vi "Query Error Status.vi"(8 "error in (no error)":errorcluster, 11 "VISA resource name":refnum<visa-resource-name>) -> (0 "error out":errorcluster, 2 "Error Status Data Message":string, 3 "VISA resource name out":refnum<visa-resource-name>)   [LabVIEW 2020, in "Stanford Research SR865.lvlib"]
doc: "Queries the Error Status register for the Error Data Register group. Essentially, it is used to observe possible invalid results."
uses:
  Stanford Research SR865.lvlib
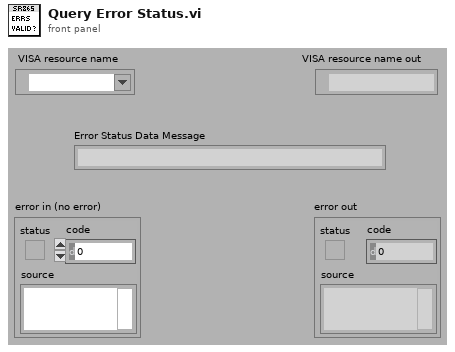
[diagram p1: front panel]
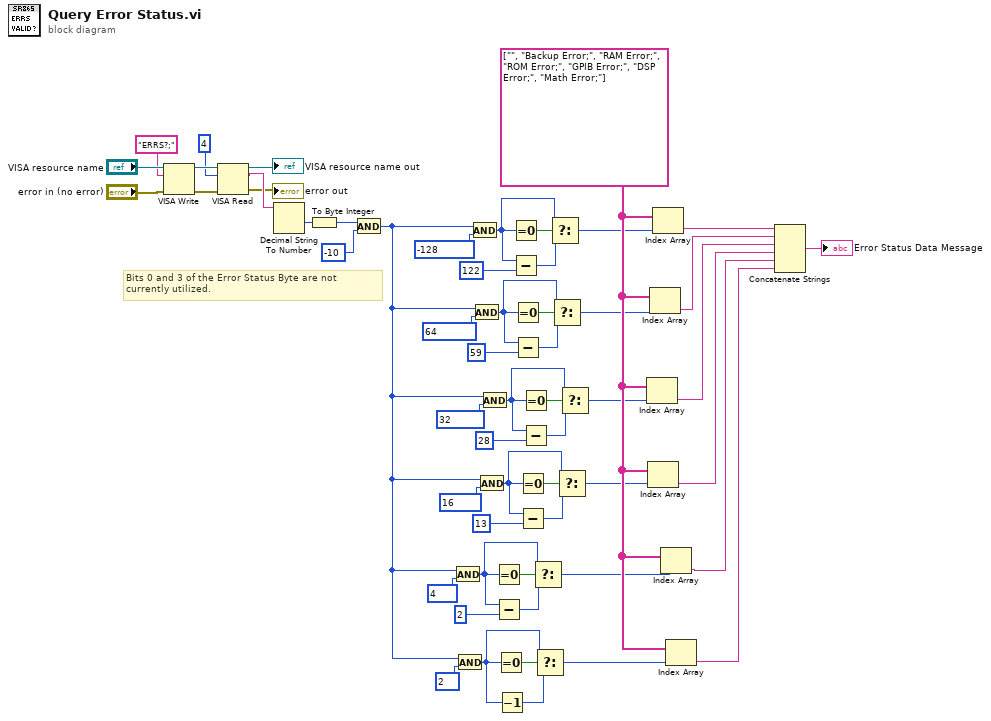
[diagram p0: block diagram]
diagram:
  w49 = string[] ["", "Backup Error;", "RAM Error;", "ROM Error;", "GPIB Error;", "DSP Error;", "Math Error;"]
  # "Bits 0 and 3 of the Error Status Byte are not currently utilized."
  n1 = VISA Write(VISA resource name="VISA resource name", write buffer="ERRS?;", error in (no error)="error in (no error)") -> (VISA resource name out=w6:refnum<visa-resource-name>, error out=w7:errorcluster)  [unwired: 1 out]
  n2 = VISA Read(VISA resource name=w6, byte count=u32 4, error in (no error)=w7) -> (VISA resource name out=→"VISA resource name out":refnum<visa-resource-name>, read buffer=w56:string, error out=→"error out":errorcluster)  [unwired: 1 out]
  n3 = Decimal String To Number(string=w56) -> (number=w3:i32)  [unwired: 2 in, 1 out]
  n4 = To Byte Integer(number=w3) -> (8bit integer=w16:i8)
  n5 = And(x=w16, y=i8 -10 ("value")) -> (x .and. y?=w53:i8)
  n6 = And(x=w53, y=i8 4) -> (x .and. y?=w43:i8)
  n7 = And(x=w53, y=i8 2) -> (x .and. y?=w1:i8)
  n8 = And(x=w53, y=i8 -128) -> (x .and. y?=w17:i8)
  n9 = And(x=w53, y=i8 64) -> (x .and. y?=w22:i8)
  n10 = And(x=w53, y=i8 16) -> (x .and. y?=w36:i8)
  n11 = And(x=w53, y=i8 32) -> (x .and. y?=w29:i8)
  n12 = Equal To 0?(x=w43) -> (x = 0?=w41:bool)
  n13 = Subtract(x=w43, y=i8 2) -> (x-y=w42:i8)
  n14 = Equal To 0?(x=w1) -> (x = 0?=w48:bool)
  n15 = Decrement(x=w1) -> (x-1=w2:i8)
  n16 = Equal To 0?(x=w17) -> (x = 0?=w13:bool)
  n17 = Subtract(x=w17, y=i8 122) -> (x-y=w14:i8)
  n18 = Equal To 0?(x=w22) -> (x = 0?=w20:bool)
  n19 = Subtract(x=w22, y=i8 59) -> (x-y=w21:i8)
  n20 = Equal To 0?(x=w36) -> (x = 0?=w34:bool)
  n21 = Subtract(x=w36, y=i8 13) -> (x-y=w35:i8)
  n22 = Equal To 0?(x=w29) -> (x = 0?=w27:bool)
  n23 = Subtract(x=w29, y=i8 28) -> (x-y=w28:i8)
  n24 = Select(t=w43, s=w41, f=w42) -> (s? t:f=w45:i8)
  n25 = Select(t=w1, s=w48, f=w2) -> (s? t:f=w50:i8)
  n26 = Select(t=w17, s=w13, f=w14) -> (s? t:f=w15:i8)
  n27 = Select(t=w22, s=w20, f=w21) -> (s? t:f=w24:i8)
  n28 = Select(t=w36, s=w34, f=w35) -> (s? t:f=w38:i8)
  n29 = Select(t=w29, s=w27, f=w28) -> (s? t:f=w31:i8)
  n30 = Index Array(array=w49, index=w31) -> (element=w32:string)
  n31 = Index Array(array=w49, index=w38) -> (element=w39:string)
  n32 = Index Array(array=w49, index=w24) -> (element=w25:string)
  n33 = Index Array(array=w49, index=w15) -> (element=w12:string)
  n34 = Index Array(array=w49, index=w45) -> (element=w46:string)
  n35 = Index Array(array=w49, index=w50) -> (element=w51:string)
  n36 = Concatenate Strings(w12, w25, w32, w39, w46, w51) -> (→"Error Status Data Message":string)
